vi "GPIO Command String.vi"(10 "Pins For Result Output (Empty Array)":i32[](array[ring]) items=["EXT1", "EXT2", "EXT3", "EXT4", "EXT5", "EXT6", "EXT7", "EXT8", "EXT9", "EXT10", "EXT11", "EXT12", "EXT13", "EXT14"]) -> (2 "Result Command String":string)   [LabVIEW 2023, in "Agilent B2900 Series.lvlib"]
doc: "Parse GPIO pins data array into comma separated string which can be recognized by SCPI Command."
uses:
  Agilent B2900 Series.lvlib
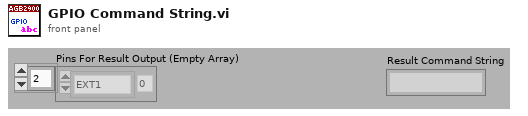
[diagram p1: front panel]
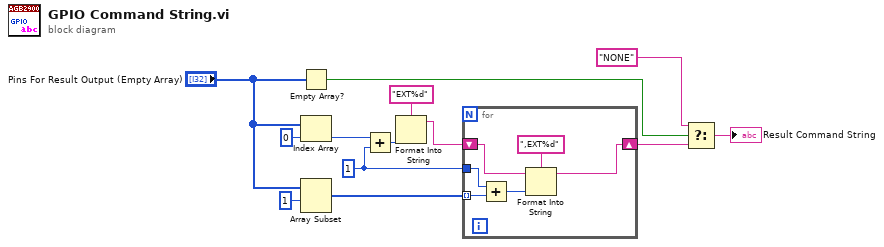
[diagram p0: block diagram]
diagram:
  w3 = 1 ("y")
  n1 = Empty Array?(array="Pins For Result Output (Empty Array)") -> (empty?=w13:bool)
  n2 = Index Array(array="Pins For Result Output (Empty Array)", index=0) -> (element=w4:i32)
  n3 = Array Subset(array="Pins For Result Output (Empty Array)", index=1) -> (w11:i32[])  [unwired: 1 in]
  n4 = Add(x=w4, y=w3) -> (x+y=w5:i32)
  n5 = Format Into String(format string="EXT%d", w5) -> (resulting string=w6:string)  [unwired: 2 in, 1 out]
  n6 = for {
    tunnel: w11 -> [w17] mode=indexing
    shift-right: [w14] -> w2
    shift-left: w6 -> [w15]
    tunnel: w3 -> [w16]
    n7 = Add(x=w16, y=w17) -> (x+y=w18:i32)
    n8 = Format Into String(format string=",EXT%d", initial string=w15, w18) -> (resulting string=w14:string)  [unwired: 1 in, 1 out]
  }
  n9 = Select(t="NONE", s=w13, f=w2) -> (s? t:f=→"Result Command String":string)
